vi "svx_Convert NaN to 0.vi"(11 "Double":dbl) -> (3 "Converted Value":dbl)   [LabVIEW 2017, in "SVX Waterfall Graph.xctl"]
uses:
  <vilib>/addons/_XControls/Waterfall Graph/SVX Waterfall Graph.xctl
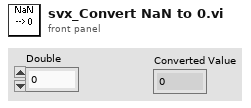
[diagram p1: front panel]
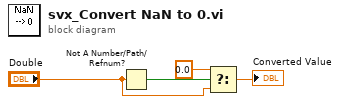
[diagram p0: block diagram]
diagram:
  n1 = Not A Number/Path/Refnum?(number/path/refnum="Double") -> (NaN/Path/Refnum?=w4:bool)
  n2 = Select(t=0.0, s=w4, f="Double") -> (s? t:f=→"Converted Value":dbl)
